vi "test img variant to data.vi"() -> ()   [LabVIEW 2013]
uses:
  <vilib>/vision/Image Controls.llb/IMAQ Image.ctl
panel:
  out "length":i32
  out "Image":T1
  out "error out":errorcluster
  out "rest of the binary string":string
  in  "data in":string
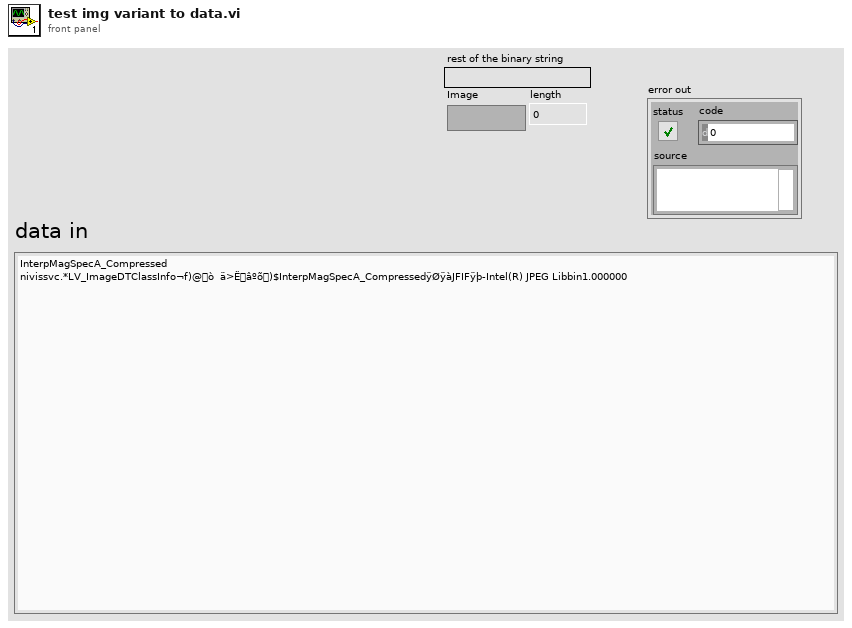
[diagram p1: front panel]
types:
  T1 = typedef "IMAQ Image.ctl" = refnum<image>
  T2 = typedef "Image Type" = u32
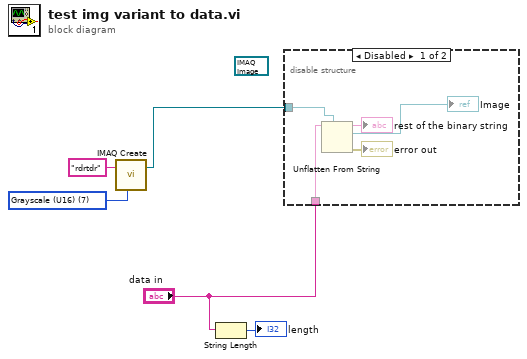
[diagram p0: block diagram]
diagram:
  w3 = T2 7 items=["Grayscale (U8)", "Grayscale (I16)", "Grayscale (SGL)", "Complex (CSG)", "RGB (U32)", "HSL (U32)", "RGB (U64)", "Grayscale (U16)"] ("Image Type")
  (unwired) T1 refnum ("Image")
  n1 = call "IMAQ Create"("Image Name"="rdrtdr", "Image Type"=w3) -> ("New Image"=w5:T1)  [unwired: 3 in, 1 out]
  n2 = String Length(string="data in") -> (length=→"length":i32)
  n3 = disable-structure shown="Disabled" {
    disable-tunnel: w5 -> [w7 _]
    disable-tunnel: "data in" -> [w6 _]
    frame Disabled {
      n4 = Unflatten From String(type=w7, binary string=w6) -> (rest of the binary string=→"rest of the binary string":string, value=→"Image":T1, error out=→"error out":errorcluster)  [unwired: 1 in, 2 out]
    }
    frame Enabled {
    }
  }
